vi "BuildMask_Motion.vi"(2 "threshold":cluster{u8, u8}(slide)={23, 255} scale=0.0..255.0, 3 "Image":T1 {"Dialogs" format="%.0b"}) -> (1 "Image":T1 {"Dialogs" format="%.0b"})   [LabVIEW 2010]
doc: "This vi will return a mask. The area inside the defined ROI is filled with 255 and the rest of the image is set to 0."
uses:
  <userlib>/ImageProcessing/QTLIB_2595_LV86/QT_Image.ctl
panel:
  # "This vi will return a mask.  The area inside the defined ROI is filled with 255 and the rest of the image is set to 0."
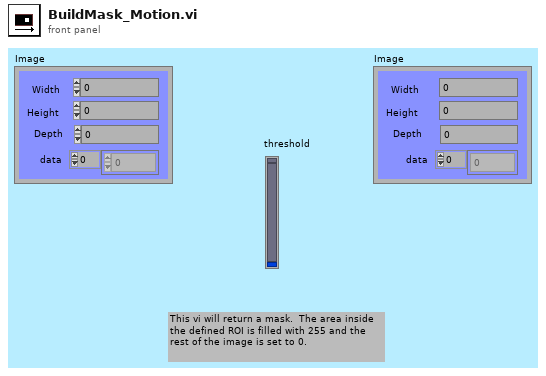
[diagram p1: front panel]
types:
  T1 = typedef "QT_Image.ctl" = cluster{"Width":i32, "Height":i32, "Depth":i32, "data":u8[], "Compressed data":u8[], "Color table":u32[], "Duration":i32, "Options":i32, "Timestamp":i32, "ID":i32, "Reserved":i32, "Dialogs":u32}
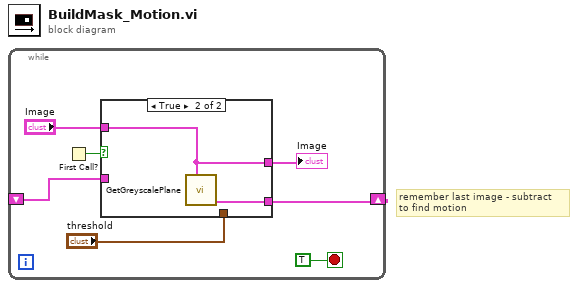
[diagram p0: block diagram]
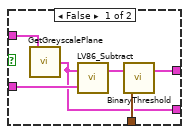
[diagram p2: hidden frame]
diagram:
  # "remember last image - subtract\nto find motion"
  n1 = while {
    shift-right: [w2] -> _
    shift-left: _ -> [w3]
    stop <- TRUE stop-if-true
    n2 = First Call?() -> (First Call?: T/F=w1:bool)
    n3 = case shown="True" w1 {
      tunnel: "threshold" -> [w13 _]
      tunnel: [w12 w15] -> w6
      tunnel: "Image" -> [w11 w15]
      tunnel: w3 -> [w10 _]
      tunnel: [w8 w14] -> w2
      frame False {
        n4 = call <userlib>:"GetGreyscalePlane.vi"("Image In"=w11) -> ("Greyscale  Out"=w8:T1)
        n5 = call <userlib>:"LV86_Subtract.vi"("Image 2"=w10, "Image"=w8) -> ("Image Out"=w9:T1)  [unwired: 1 in]
        n6 = call <userlib>:"BinaryThreshold.vi"("threshold"=w13, "Image In"=w9) -> ("Image Out"=w12:T1)  [unwired: 1 in]
      }
      frame True {
        n7 = call <userlib>:"GetGreyscalePlane.vi"("Image In"=w15) -> ("Greyscale  Out"=w14:T1)
      }
    }
    "Image" <- w6
  }
